vi "Metadata - table.vi"(8 "error in (no error)":errorcluster, 10 "Table in":string, 11 "sqlite in":refnum<class "sqlite3.lvclass">) -> (0 "error out":errorcluster, 2 "PRAGMA table info":string[][](array[string]), 3 "sqlite out":refnum<class "sqlite3.lvclass">)   [LabVIEW 2020, in "sqlite3.lvlib" / "sqlite3.lvclass"]
uses:
  sqlite3.lvclass
  sqlite3.lvclass/sqlite3.ctl
  db layer/compound/Execute SQL.vi
  sqlite/VIs/open v2.vi
  sqlite/VIs/prepare v2.vi
  sqlite/VIs/step.vi
  sqlite/VIs/column count.vi
  db layer/compound/Column.vi
  db layer/compound/Resolve Result Type.vi
  sqlite/VIs/finalize.vi
  sqlite/VIs/close v2.vi
  sqlite/subvi/Error Converter (ErrCode or Status).vi
  sqlite/VIs/column text.vi
  sqlite/VIs/column bytes.vi
  sqlite/VIs/column blob.vi
  db layer/utilities/MoveBlock.vi
  sqlite/VIs/column type.vi
  sqlite/VIs/errstr.vi
  sqlite3.lvlib
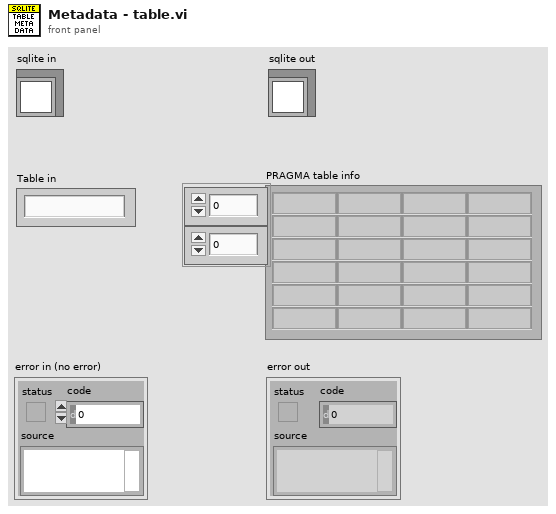
[diagram p1: front panel]
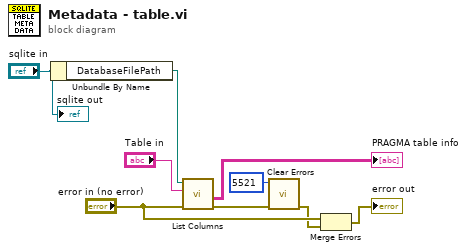
[diagram p0: block diagram]
diagram:
  n1 = Unbundle By Name("sqlite in") -> ("DatabaseFilePath"=w7:path)
  n2 = call "List Columns.vi"("error in (no error)"="error in (no error)", "Table name"="Table in", "database in"=w7) -> ("error out"=w5:errorcluster, "PRAGMA table info"=→"PRAGMA table info":string[][])  [unwired: 5 in, 2 out]
  n3 = call <vilib>:"Clear Errors.vi"("error in (no error)"=w5, "specific error code to clear (0: all)"=5521) -> ("error out"=w2:errorcluster)  [unwired: 4 in, 1 out]
  n4 = Merge Errors("error in (no error)", w2) -> (→"error out":errorcluster)
  "sqlite out" <- "sqlite in"
